vi "insertPackageData.vi"(7 "path in":path=path "C:/dev/Hexagon-VTD-Custom-Device/Libraries/VC.dll", 8 "error in (no error)":errorcluster, 9 "packageData":u8[](array[numeric]), 10 "packageID":u16, 11 "builderHandle in":u64) -> (0 "error out":errorcluster, 2 "packageData":u8[](array[numeric]), 3 "builderHandle out":u64)   [LabVIEW 2023, in "RDB.lvlib"]
uses:
  RDB.lvlib
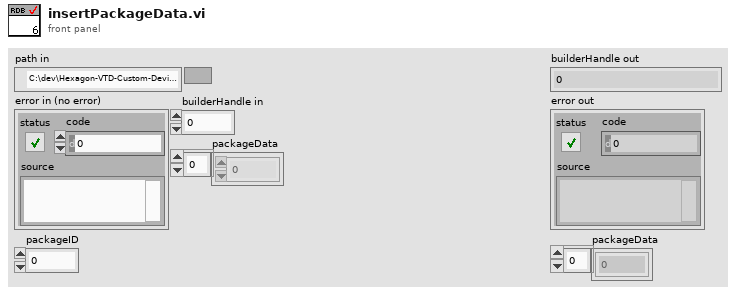
[diagram p1: front panel]
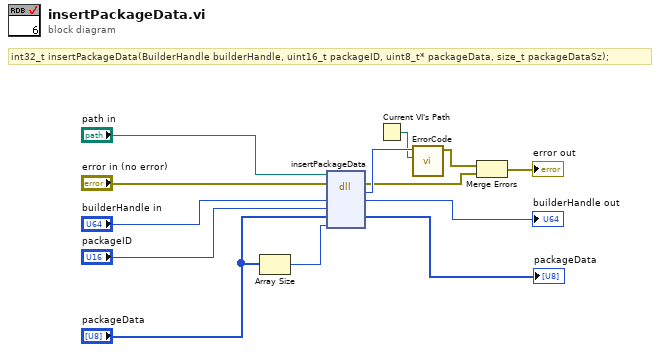
[diagram p0: block diagram]
diagram:
  # "int32_t insertPackageData(BuilderHandle builderHandle, uint16_t packageID, uint8_t* packageData, size_t packageDataSz);"
  n1 = Array Size(array="packageData") -> (size(s)=w2:i32)
  n2 = dll-call lib="C:/dev/Hexagon-VTD-Custom-Device/Libraries/libVC.dll" fn="insertPackageData"(path in="path in", error in="error in (no error)", "builderHandle"="builderHandle in", "packageID"="packageID", "packageData"="packageData", "packageDataSz"=w2) -> (error out=w8:errorcluster, "return type"=w10:i32, "builderHandle"=→"builderHandle out":u64, "packageData"=→"packageData":u8[])  [unwired: 3 in, 1 out]
  n3 = Current VI's Path() -> (path=w5:path)
  n4 = call "ErrorCode.vi"("parent VI path"=w5, "return type"=w10) -> ("error out"=w9:errorcluster)  [unwired: 9 in]
  n5 = Merge Errors(w9, w8) -> (→"error out":errorcluster)
